vi "n set scanner delays.vi"(7 "polydelay":u16, 8 "error in (no error)":errorcluster, 9 "markdelay":u16, 10 "jumpdelay":u16, 11 "n":u16) -> (0 "error out":errorcluster)   [LabVIEW 2015, in "SCANalone4x64.lvlib"]
doc: "__declspec(dllimport) void __stdcall n_set_scanner_delays(unsigned short n, unsigned short jumpdelay, unsigned short markdelay, unsigned short polydelay);"
uses:
  <userlib>/SCANalone4x64/SCANalone4x64.lvlib
  <userlib>/SCANalone4x64/SCANalone4x64.dll
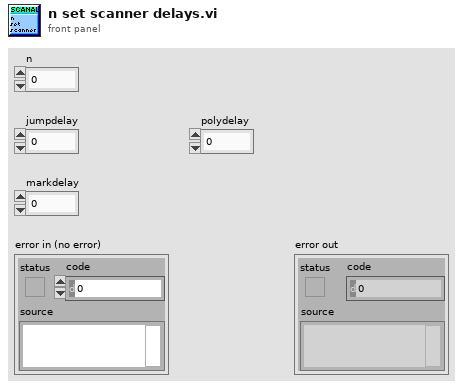
[diagram p1: front panel]
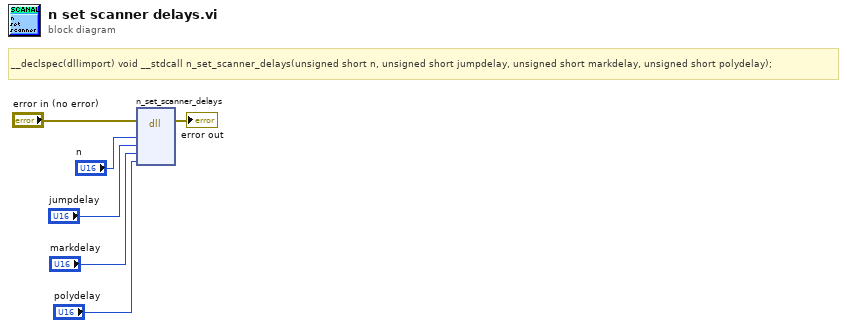
[diagram p0: block diagram]
diagram:
  # "__declspec(dllimport) void __stdcall n_set_scanner_delays(unsigned short n, unsigned short jumpdelay, unsigned short markdelay, unsigned short polydelay);"
  n1 = dll-call lib="C:/Program Files/National Instruments/LabVIEW 2015/user.lib/SCANalone4x64/SCANalone4x64.*" fn="n_set_scanner_delays"(error in="error in (no error)", "n"="n", "jumpdelay"="jumpdelay", "markdelay"="markdelay", "polydelay"="polydelay") -> (error out=→"error out":errorcluster)  [unwired: 7 in, 1 out]
